vi "DataRIC2NumConv.vi"(11 "Cluster":cluster{string, string, string}) -> (0 "Data":u8[](array[numeric]), 3 "Numeric":u8)   [LabVIEW 2017]
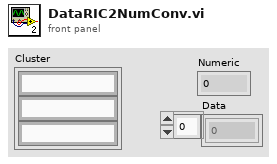
[diagram p1: front panel]
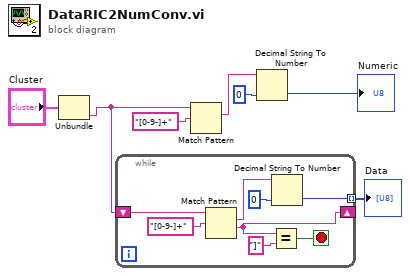
[diagram p0: block diagram]
diagram:
  n1 = Unbundle("Cluster") -> (w2:string)  [unwired: 2 out]
  n2 = while {
    shift-right: [w12] -> _
    shift-left: w2 -> [w15]
    tunnel: [w9] -> w1 mode=indexing
    stop <- w11 stop-if-true
    n3 = Match Pattern(string=w15, regular expression="[0-9-]+") -> (match substring=w10:string, after substring=w12:string)  [unwired: 1 in, 2 out]
    n4 = Equal?(x=w12, y="]") -> (x = y?=w11:bool)
    n5 = Decimal String To Number(string=w10, default (0L)=u8 0 ("default (0 I32)")) -> (number=w9:u8)  [unwired: 1 in, 1 out]
  }
  "Data" <- w1
  n6 = Match Pattern(string=w2, regular expression="[0-9-]+") -> (match substring=w4:string)  [unwired: 1 in, 3 out]
  n7 = Decimal String To Number(string=w4, default (0L)=u8 0 ("default (0 I32)")) -> (number=→"Numeric":u8)  [unwired: 1 in, 1 out]
